vi "Read Test Param.vi"(8 "error in (no error)":errorcluster, 11 "Test Switch Init Parameters in":refnum<class "Test Switch Init Parameters.lvclass">) -> (0 "error out":errorcluster, 2 "Param 1":string, 3 "Test Switch Init Parameters out":refnum<class "Test Switch Init Parameters.lvclass">)   [LabVIEW 2017, in "Test Switch Init Parameters.lvclass"]
uses:
  Test Switch Init Parameters.lvclass
  Test Switch Init Parameters.lvclass/Test Switch Init Parameters.ctl
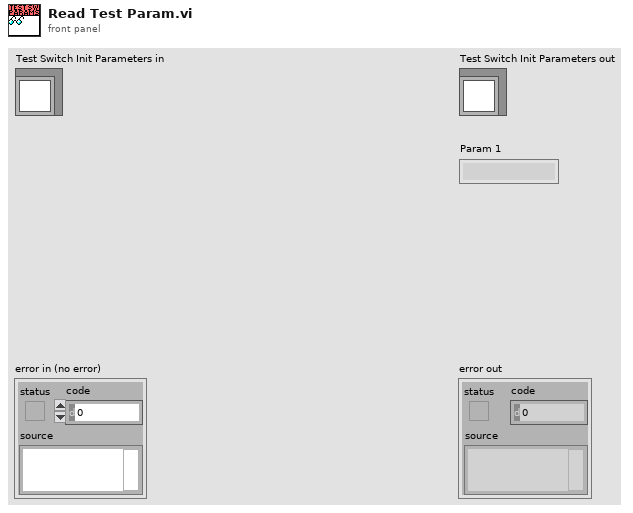
[diagram p1: front panel]
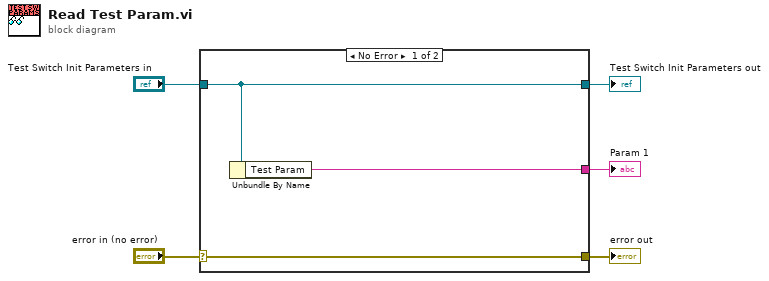
[diagram p0: block diagram]
diagram:
  n1 = case shown="No Error" "error in (no error)" {
    selector: "error in (no error)" -> [w8 w9]
    tunnel: [w8 w9] -> w4
    tunnel: [w7 w10] -> w2
    tunnel: "Test Switch Init Parameters in" -> [w7 w10]
    tunnel: [w6 _] -> w1
    frame No Error {
      n2 = Unbundle By Name(w7) -> ("Test Param"=w6:string)
    }
    frame Error {
    }
  }
  "error out" <- w4
  "Test Switch Init Parameters out" <- w2
  "Param 1" <- w1
